vi "Tool - FP size and position.vi"(0 "vi ref (this vi)":refnum<vi>, 2 "FP Origin (0,0)":cluster{"Horizontal":i16, "Vertical":i16}, 3 "Window Size(No Resize)":cluster{"Width":i16, "Height":i16}, 4 "Pane Index":i32, 5 "error in (no error)":errorcluster, 6 "Move Window (F)":bool, 7 "SetAllPanes? (T)":bool=TRUE, 8 "Window Origin (0,0)":cluster{"Left":i16, "Top":i16}, 9 "Close Ref? (T)":bool=TRUE) -> (14 "dup ref":refnum<vi>, 19 "error out":errorcluster)   [LabVIEW 2015, in "QuickVIew.lvlib" / "TLB`_Dependencies.lvlib"]
doc: "Resizes the window of the parent VI and sets the origin to 0,0. Intended to be done at initialization to properly orient and size the front panel.TLB Prime - Application Template 1.3.0.24\nNorm Kirchner, NI Systems Engineering - NI\nCopyright (c) 2014, NI"
uses:
  TLB`_Dependencies.lvlib
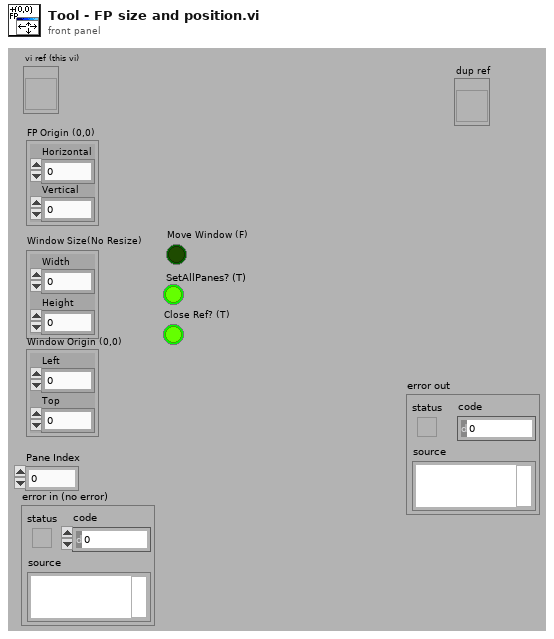
[diagram p1: front panel]
types:
  T1 = typedef "LVRectTypeDef.ctl" = cluster{"Left":i16, "Top":i16, "Right":i16, "Bottom":i16}
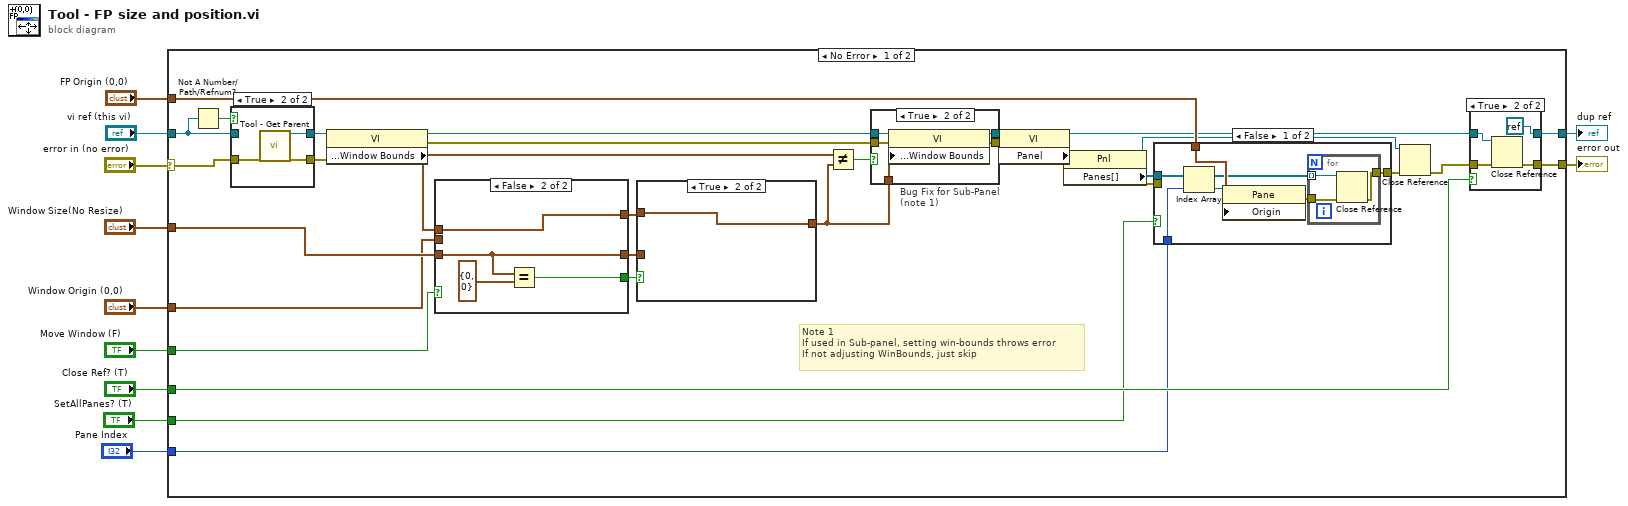
[diagram p0: block diagram]
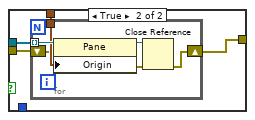
[diagram p3: hidden frame]
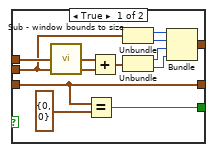
[diagram p4: hidden frame]
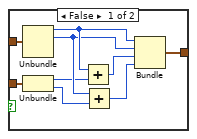
[diagram p5: hidden frame]
diagram:
  n1 = case shown="No Error" "error in (no error)" {
    selector: "error in (no error)" -> [w40 w107]
    tunnel: "vi ref (this vi)" -> [w41 w108]
    tunnel: [w36 w108] -> w10
    tunnel: [w38 w107] -> w9
    tunnel: "FP Origin (0,0)" -> [w22 _]
    tunnel: "Window Size(No Resize)" -> [w35 _]
    tunnel: "Close Ref? (T)" -> [w37 _]
    tunnel: "Window Origin (0,0)" -> [w33 _]
    tunnel: "Move Window (F)" -> [w31 _]
    tunnel: "SetAllPanes? (T)" -> [w16 _]
    tunnel: "Pane Index" -> [w15 _]
    frame No Error {
      # "Note 1\nIf used in Sub-panel, setting win-bounds throws error\nIf not adjusting WinBounds, just skip"
      n2 = Not A Number/Path/Refnum?(number/path/refnum=w41) -> (NaN/Path/Refnum?=w43:bool)
      n3 = case shown="True" w43 {
        tunnel: [w103 w106] -> w42
        tunnel: w41 -> [w103 _]
        tunnel: w40 -> [w102 w105]
        tunnel: [w102 w104] -> w39
        frame False {
        }
        frame True {
          n4 = call "Tool - Get Parent.vi"("error in (no error)"=w105) -> ("VI Refnum"=w106:refnum<vi>, "error out"=w104:errorcluster)  [unwired: 2 in, 15 out]
        }
      }
      n5 = property class="VI"(reference=w42, error in=w39) -> (reference out=w25:refnum<vi>, error out=w26:errorcluster, "Front Panel Window:Window Bounds"=w13:T1)
      n6 = case shown="False" w31 {
        tunnel: w35 -> [w70 w82]
        tunnel: [w80 w84] -> w34
        tunnel: w33 -> [w71 _]
        tunnel: [w73 w83] -> w32
        tunnel: w13 -> [w72 w83]
        tunnel: [w70 w82] -> w30
        frame True {
          n7 = call "Sub - window bounds to size.vi"("Bounds"=w72) -> ("Size"=w79:cluster{"Width":i16, "Height":i16})
          n8 = Equal?(x=w70, y=cluster{"Width (800)":i16, "Height (600)":i16} {"Width (800)"=0, "Height (600)"=0} ("Window Size (800,600)")) -> (x = y?=w80:bool)
          n9 = Add(x=w79, y=w71) -> (x+y=w78:cluster{i16, i16})
          n10 = Unbundle(w71) -> ("Left"=w77:i16, "Top"=w76:i16)
          n11 = Unbundle(w78) -> (w75:i16, w74:i16)
          n12 = Bundle("Left"=w77, "Top"=w76, w75, w74) -> (w73:cluster{"Left":i16, "Top":i16, i16, i16})  [unwired: 1 out]
        }
        frame False {
          n13 = Equal?(x=w82, y=cluster{"Width (800)":i16, "Height (600)":i16} {"Width (800)"=0, "Height (600)"=0} ("Window Size (800,600)")) -> (x = y?=w84:bool)
        }
      }
      n14 = case shown="True" w34 {
        tunnel: w32 -> [w91 w95]
        tunnel: w30 -> [w88 _]
        tunnel: [w89 w95] -> w14
        frame False {
          n15 = Unbundle(w91) -> ("Left"=w94:i16, "Top"=w93:i16)  [unwired: 2 out]
          n16 = Unbundle(w88) -> ("Width"=w87:i16, "Height"=w86:i16)
          n17 = Add(x=w94, y=w87) -> (x+y=w92:i16)
          n18 = Add(x=w93, y=w86) -> (x+y=w90:i16)
          n19 = Bundle("Left"=w94, "Top"=w93, w92, w90) -> (w89:cluster{"Left":i16, "Top":i16, i16, i16})  [unwired: 1 out]
        }
        frame True {
        }
      }
      n20 = Not Equal?(x=w13, y=w14) -> (x != y?=w12:bool)
      n21 = case "Bug Fix for Sub-Panel (note 1)" shown="True" w12 {
        tunnel: w26 -> [w44 w50]
        tunnel: w25 -> [w45 w49]
        tunnel: [w44 w48] -> w24
        tunnel: [w45 w47] -> w23
        tunnel: w14 -> [_ w46]
        frame False {
        }
        frame True {
          n22 = property class="VI"(reference=w49, error in=w50, "Front Panel Window:Window Bounds"=w46) -> (reference out=w47:refnum<vi>, error out=w48:errorcluster)
        }
      }
      n23 = property class="VI"(reference=w23, error in=w24) -> (reference out=w18:refnum<vi>, error out=w27:errorcluster, "Panel"=w29:refnum<vi>)
      n24 = property class="Pnl"(reference=w29, error in=w27) -> (reference out=w20:refnum<vi>, error out=w21:errorcluster, "Panes[]"=w28:refnum<vi>[])
      n25 = case shown="False" w16 {
        tunnel: w28 -> [w53 w63]
        tunnel: w22 -> [w54 w62]
        tunnel: w21 -> [_ w61]
        tunnel: [w51 w60] -> w19
        tunnel: w15 -> [w56 _]
        frame False {
          n26 = Index Array(array=w53, index=w56) -> (element=w55:refnum<vi>)
          n27 = property class="Pane"(reference=w55, "Origin"=w54) -> (error out=w52:errorcluster)  [unwired: 1 in, 1 out]
          n28 = for {
            tunnel: w53 -> [w59] mode=indexing
            tunnel: w52 -> [w58]
            tunnel: [w57] -> w51
            n29 = Close Reference(reference=w59, error in (no error)=w58) -> (error out=w57:errorcluster)
          }
        }
        frame True {
          n30 = for {
            tunnel: w63 -> [w69] mode=indexing
            tunnel: w62 -> [w66]
            shift-right: [w65] -> w60
            shift-left: w61 -> [w64]
            n31 = property class="Pane"(reference=w69, error in=w64, "Origin"=w66) -> (reference out=w68:refnum<vi>, error out=w67:errorcluster)
            n32 = Close Reference(reference=w68, error in (no error)=w67) -> (error out=w65:errorcluster)
          }
        }
      }
      n33 = Close Reference(reference=w20, error in (no error)=w19) -> (error out=w17:errorcluster)
      n34 = case shown="True" w37 {
        tunnel: w18 -> [w97 w99]
        tunnel: w17 -> [w96 w101]
        tunnel: [w96 w100] -> w38
        tunnel: [w97 refnum<k0> refnum] -> w36
        frame False {
        }
        frame True {
          n35 = Close Reference(reference=w99, error in (no error)=w101) -> (error out=w100:errorcluster)
        }
      }
    }
    frame Error {
    }
  }
  "dup ref" <- w10
  "error out" <- w9
